vi "WinCI Get Version.vi"(8 "error in (no error)":errorcluster) -> (0 "error out":errorcluster, 1 "minor revision":u16, 2 "major revision":u16)   [LabVIEW 2017, in "NI_SCC_WinCI.lvlib"]
uses:
  <vilib>/SourceControl/Providers/WinCI/NI_SCC_WinCI.lvlib
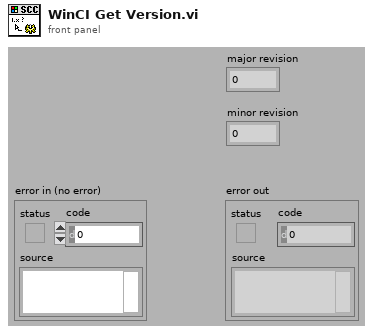
[diagram p1: front panel]
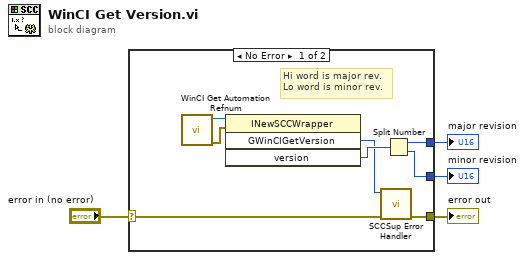
[diagram p0: block diagram]
diagram:
  n1 = case shown="No Error" "error in (no error)" {
    selector: "error in (no error)" -> [w12 w13]
    tunnel: [w11 w13] -> w3
    tunnel: [w10 _] -> w2
    tunnel: [w9 _] -> w1
    frame No Error {
      # "Hi word is major rev.\nLo word is minor rev."
      n2 = call <vilib>:"WinCI Get Automation Refnum.vi"() -> ("error out"=w6:errorcluster, "automation refnum"=w5:refnum<k7>)  [unwired: 10 out]
      n3 = invoke class="INewSCCWrapper" method="GWinCIGetVersion"(reference=w5, error in=w6) -> ("GWinCIGetVersion"=w7:i32, "version"=w8:i32)  [unwired: 2 in, 2 out]
      n4 = call <vilib>:"SCCSup Error Handler.vi"("error in (no error)"=w12, "scc error code"=w7) -> ("error out"=w11:errorcluster)  [unwired: 2 in, 7 out]
      n5 = Split Number(x=w8) -> (hi(x)=w10:u16, lo(x)=w9:u16)
    }
    frame Error {
    }
  }
  "error out" <- w3
  "major revision" <- w2
  "minor revision" <- w1
